vi "Periodic Tasks.vi"(8 "error in":errorcluster) -> ()   [LabVIEW 2017]
doc: "This VI runs in parallel to other tasks. It can contain as many user-defined periodic loops as you need. These can carry out PID or other sorts of timed response."
uses:
  <vilib>/Rock Robotics/WPI/Utilities/WPI_GetSetVariantRefNum.vi
  <vilib>/Rock Robotics/Network Tables/NT Write Number.vi
panel:
  in  "Reset Encoder?":bool
  out "Encoder Distance":dbl
  out "Encoder Rate (distance/sec)":dbl
  out "Encoder Alarm Status":string
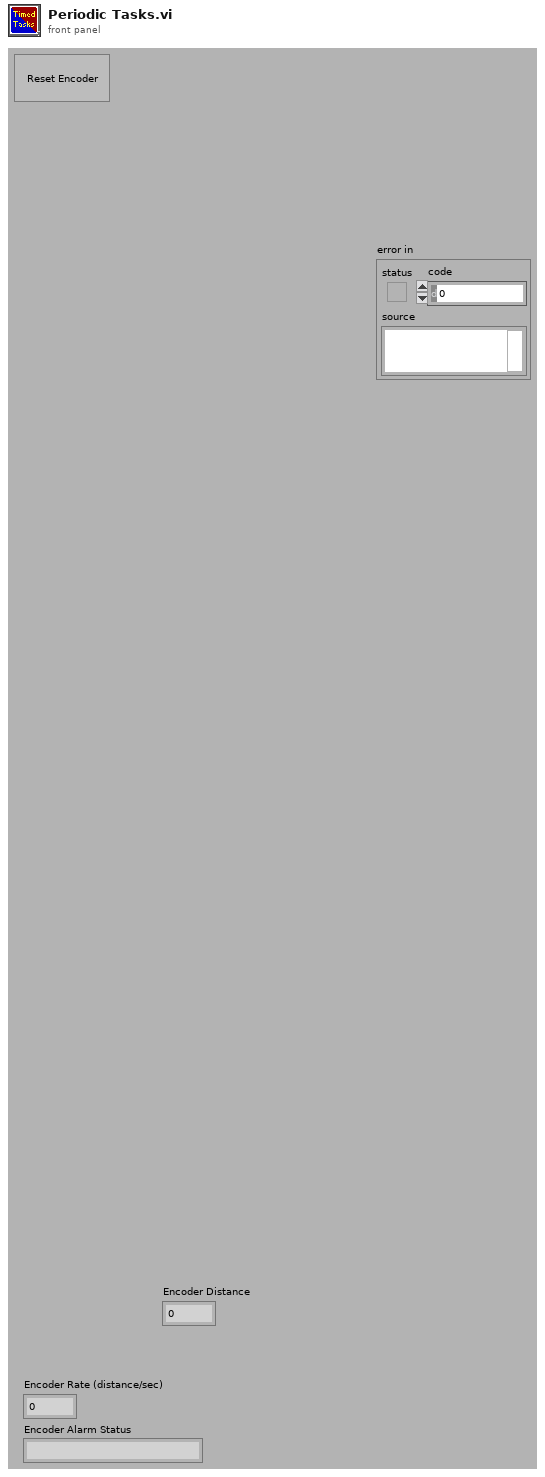
[diagram p1: front panel]
types:
  T1 = typedef "WPI_JoystickDevRef.ctl" = cluster{"Device":T2}
  T2 = typedef "WPI_JoystickDeviceEnum.ctl" = enum16{"USB 0", "USB 1", "USB 2", "USB 3", "USB 4", "USB 5"}
  T3 = typedef "WPI_RobotDriveDevRef.ctl" = cluster{"DevStatus":errorcluster, "Motors[]":T4[], "Square Inputs":bool, "Max Output":dbl}
  T4 = typedef "WPI_MotorControlDeviceRef.ctl" = cluster{"DeviceStatus":errorcluster, "Type":T5, "PWM":cluster{"PWM Channel":T6, "DeadBand":T7}, "CAN":cluster{"Device Number":u8, "SetOutput VI Ref":variant, "GetOutput VI Ref":variant, "Enable VI Ref":variant, "Disable VI Ref":variant, "Data":variant}, "Invert":bool, "DIO PWM":cluster{"PWM \"Enable\" Channel":T6, "DIOChannel":T8, "PWM Rate":dbl}}
  T5 = typedef "WPI_MotorControlType.ctl" = enum16{"PWM", "CAN", "DIO PWM"}
  T6 = typedef "FPGA_DIOPWMChannel.ctl" = enum8{"PWM 0", "PWM 1", "PWM 2", "PWM 3", "PWM 4", "PWM 5", "PWM 6", "PWM 7", "PWM 8", "PWM 9", "PWM MXP 0", "PWM MXP 1", "PWM MXP 2", "PWM MXP 3", "PWM MXP 4", "PWM MXP 5", "PWM MXP 6", "PWM MXP 7", "PWM MXP 8", "PWM MXP 9", "Invalid"}
  T7 = typedef "WPI_PWMDeadband.ctl" = cluster{"Name":string, "maxPositivePwm":i32, "minPositivePwm":i32, "centerPwm":i32, "maxNegativePwm":i32, "minNegativePwm":i32, "angularRange":u16}
  T8 = typedef "FPGA_DIOChannel.ctl" = enum8{"DIO 0", "DIO 1", "DIO 2", "DIO 3", "DIO 4", "DIO 5", "DIO 6", "DIO 7", "DIO 8", "DIO 9", "DIO MXP 0", "DIO MXP 1", "DIO MXP 2", "DIO MXP 3", "DIO MXP 4", "DIO MXP 5", "DIO MXP 6", "DIO MXP 7", "DIO MXP 8", "DIO MXP 9", "DIO MXP 10", "DIO MXP 11", "DIO MXP 12", "DIO MXP 13", "DIO MXP 14", "DIO MXP 15", "SPI Port CS1", "SPI Port CS2", "SPI Port CS3", "SPI Port MISO", "SPI Port MOSI", "Invalid"}
  T9 = typedef "WPI_EncoderDevRef.ctl" = cluster{"DevStatus":errorcluster, "EncoderIndex":T10, "CounterIndex":T11, "DistancePerCount":dbl, "Decoding Type":T12}
  T10 = typedef "FPGA_EncoderIdx.ctl" = enum8{"Enc 0", "Enc 1", "Enc 2", "Enc 3", "Enc 4", "Enc 5", "Enc 6", "Enc 7", "Invalid"}
  T11 = typedef "FPGA_CounterCtrSystemIndex.ctl" = enum8{"Ctr 0", "Ctr 1", "Ctr 2", "Ctr 3", "Ctr 4", "Ctr 5", "Ctr 6", "Ctr 7", "Invalid"}
  T12 = typedef "WPI_EncoderType.ctl" = enum16{"1x", "2x", "4x"}
  T13 = cluster{"JoystickDevRef":T1, "RobotDriveDevRef":T3}
  T14 = typedef "WPI_GyroDevRef.ctl" = cluster{"DevStatus":errorcluster, "Analog Channel":T15, "Gain (VoltsPerDegree/Second)":dbl, "Gyro Type":enum16{"Analog", "XRS450"}, "Handle":i32, "SPI Bus":T16, "Device Found":bool, "Sample Rate":dbl, "Calibrate On Open":bool, "Offset":dbl}
  T15 = typedef "FPGA_AIChannel.ctl" = enum8{"AI 0", "AI 1", "AI 2", "AI 3", "AI MXP 0", "AI MXP 1", "AI MXP 2", "AI MXP 3", "Invalid"}
  T16 = typedef "spi_bus.ctl" = enum16{"SPI On-Board, CS0", "SPI On-Board, CS1", "SPI On-Board, CS2", "SPI On-Board, CS3", "SPI MXP", "Invalid"}
  T17 = cluster{"Axes[0]":dbl, "Axes[1]":dbl, "Axes[2]":dbl, "Axes[3]":dbl, "Axes[4]":dbl, "Axes[5]":dbl, "Axes[6]":dbl, "Axes[7]":dbl, "Axes[8]":dbl}
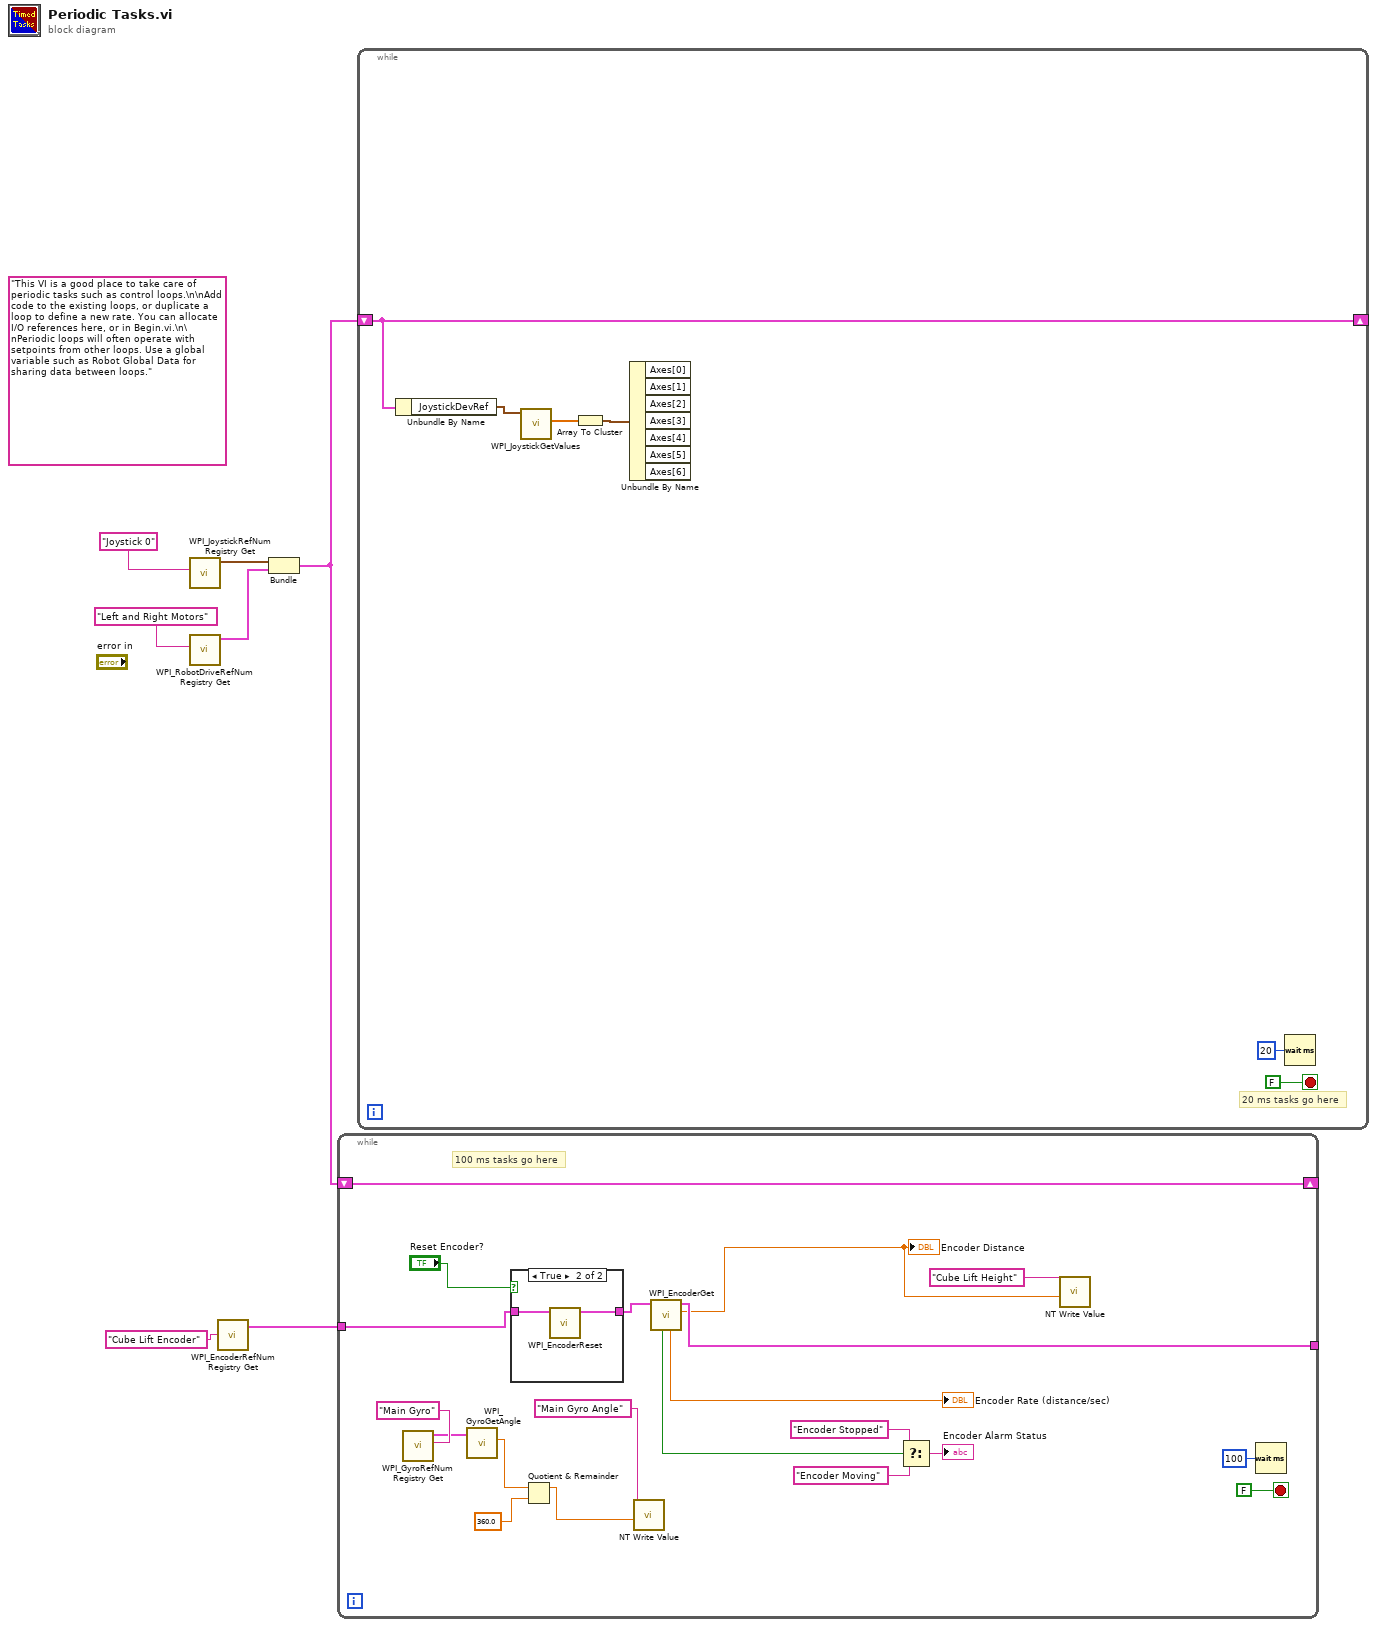
[diagram p0: block diagram]
diagram:
  (unwired) "This VI is a good place to take care of periodic tasks such as control loops.\n\nAdd code to the existing loops, or duplicate a loop to define a new rate. You can allocate I/O references here, or in Begin.vi.\n\nPeriodic loops will often operate with setpoints from other loops. Use a global variable such as Robot Global Data for sharing data between loops."
  n1 = call <vilib>:"WPI_JoystickRefNum Registry Get.vi"("refnum name"="Joystick 0") -> ("JoystickDevRef"=w5:T1)  [unwired: 1 in, 9 out]
  n2 = call <vilib>:"WPI_RobotDriveRefNum Registry Get.vi"("refnum name"="Left and Right Motors") -> ("RobotDriveDevRef"=w4:T3)  [unwired: 1 in, 9 out]
  n3 = call <vilib>:"WPI_EncoderRefNum Registry Get.vi"("refnum name"="Cube Lift Encoder") -> ("EncoderDevRef"=w1:T9)  [unwired: 9 in, 1 out]
  n4 = Bundle("JoystickDevRef"=w5, "RobotDriveDevRef"=w4) -> (w3:T13)  [unwired: 1 out]
  n5 = while {
    shift-right: [w25] -> _
    shift-left: w3 -> [w25]
    tunnel: [w20] -> _
    tunnel: w1 -> [w19]
    stop <- FALSE stop-if-true
    # "100 ms tasks go here"
    n6 = call <vilib>:"WPI_GyroRefNum Registry Get.vi"("refnum name"="Main Gyro") -> ("GyroDevRef"=w12:T14)  [unwired: 9 in, 1 out]
    n7 = call <vilib>:"WPI_GyroGetAngle.vi"("GyroDevRef"=w12) -> ("Angle"=w10:dbl)  [unwired: 6 in, 4 out]
    n8 = case shown="True" "Reset Encoder?" {
      tunnel: w19 -> [w28 w30]
      tunnel: [w28 w29] -> w21
      frame False {
      }
      frame True {
        n9 = call <vilib>:"WPI_EncoderReset.vi"("EncoderDevRef"=w30) -> ("EncoderDevRef"=w29:T9)  [unwired: 1 in, 9 out]
      }
    }
    n10 = Quotient & Remainder(x=w10, y=360.0) -> (x-y*floor(x/y)=w9:dbl)  [unwired: 1 out]
    n11 = call-poly <vilib>:"NT Write Value.vi"("Numeric"=w9, "Name"="Main Gyro Angle") -> ()  [unwired: 9 in, 1 out]
    n12 = call <vilib>:"WPI_EncoderGet.vi"("EncoderDevRef"=w21) -> ("Distance"=w15:dbl, "EncoderDevRef"=w20:T9, "Rate"=→"Encoder Rate (distance/sec)":dbl, "Stopped"=w17:bool)  [unwired: 1 in, 6 out]
    "Encoder Distance" <- w15
    n13 = Select(t="Encoder Stopped", s=w17, f="Encoder Moving") -> (s? t:f=→"Encoder Alarm Status":string)
    n14 = call-poly <vilib>:"NT Write Value.vi"("Numeric"=w15, "Name"="Cube Lift Height") -> ()  [unwired: 9 in, 1 out]
    n15 = Wait (ms)(milliseconds to wait=u32 100) -> ()  [unwired: 1 out]
  }
  n16 = while {
    shift-right: [w34] -> _
    shift-left: w3 -> [w34]
    stop <- FALSE stop-if-true
    # "20 ms tasks go here"
    n17 = Unbundle By Name(w34) -> ("JoystickDevRef"=w33:T1)
    n18 = call <vilib>:"WPI_JoystickGetValues.vi"("JoystickDevRef"=w33) -> ("Axes"=w31:dbl[])  [unwired: 6 in, 4 out]
    n19 = Array To Cluster(array=w31) -> (cluster=w32:T17)
    n20 = Unbundle By Name(w32) -> ()  [unwired: 7 out]
    n21 = Wait (ms)(milliseconds to wait=u32 20) -> ()  [unwired: 1 out]
  }
